vi "S2C_IMAGE_Proc_PassFail.vi"(8 "Error In":errorcluster, 11 "ImagePath":path) -> (0 "Error Out":errorcluster, 3 "Result":string)   [LabVIEW 2015]
panel:
  in  "Submit":bool
  in  "Blemesh":bool
  in  "Chip":bool
  in  "Dent":bool
  in  "Scratch":bool
  out "Image":picture
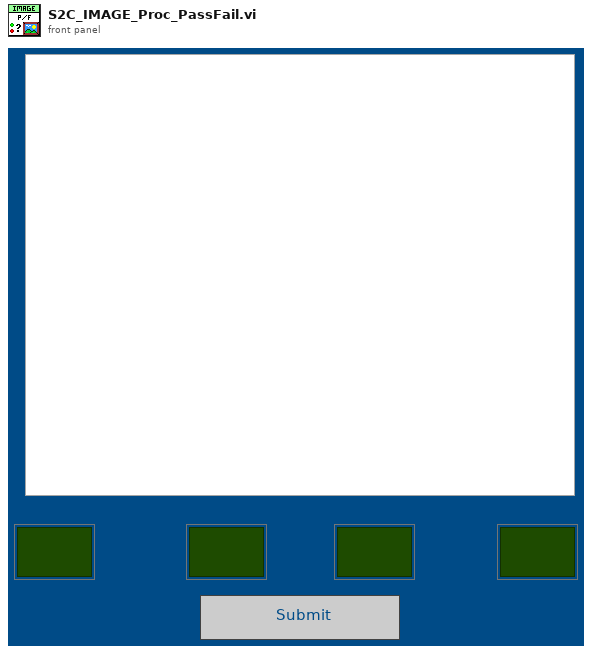
[diagram p1: front panel]
types:
  T1 = cluster{"Left":i16, "Top":i16, "Right":i16, "Bottom":i16}
  T2 = enum32{"Invalid", "Standard", "Closed", "Hidden", "Minimized", "Maximized"}
  T3 = typedef "imagedata.ctl" = cluster{"image type":i32, "image depth":i32, "image":u8[], "mask":u8[], "colors":u32[], "Rectangle":cluster{"left":i16, "top":i16, "right":i16, "bottom":i16}}
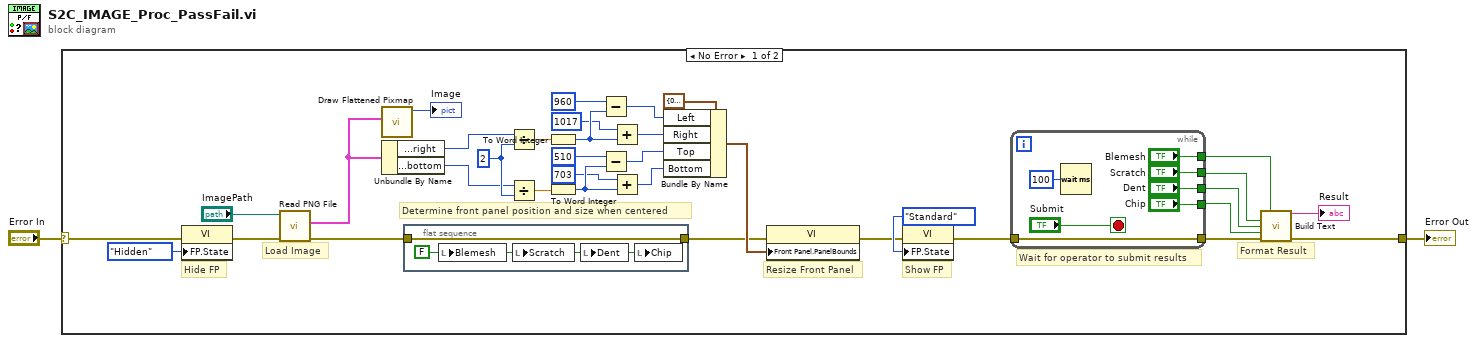
[diagram p0: block diagram]
diagram:
  n1 = case shown="No Error" "Error In" {
    selector: "Error In" -> [w34 w47]
    tunnel: [w26 w47] -> w1
    frame No Error {
      w28 = i16 2 ("y")
      # "Format Result"
      # "Show FP"
      # "Resize Front Panel"
      # "Determine front panel position and size when centered"
      # "Hide FP"
      # "Wait for operator to submit results"
      # "Load Image"
      n2 = property class="VI"(error in=w34, "FP.State"=T2."Hidden" ("Front Panel Window:State")) -> (error out=w32:errorcluster)  [unwired: 1 in, 1 out]
      n3 = call <vilib>:"Read PNG File.vi"("error in (no error)"=w32, "path to PNG file"="ImagePath") -> ("error out"=w4:errorcluster, "image data"=w35:T3)  [unwired: 7 in, 1 out]
      n4 = call <vilib>:"Draw Flattened Pixmap.vi"("image data"=w35) -> ("new picture"=→"Image":picture)  [unwired: 8 in]
      n5 = Unbundle By Name(w35) -> ("Rectangle.right"=w7:i16, "Rectangle.bottom"=w6:i16)
      n6 = flat-sequence {
        tunnel: w4 -> [w39]
        tunnel: [w39] -> w3
        frame #0 {
          w38 = FALSE ("Blemesh")
          n7 = local write "Blemesh"(w38) -> ()
          n8 = local write "Scratch"(w38) -> ()
          n9 = local write "Dent"(w38) -> ()
          n10 = local write "Chip"(w38) -> ()
        }
      }
      n11 = Divide(x=w7, y=w28) -> (x/y=w9:dbl)
      n12 = Divide(x=w6, y=w28) -> (x/y=w8:dbl)
      n13 = To Word Integer(number=w9) -> (16bit integer=w19:i16)
      n14 = To Word Integer(number=w8) -> (16bit integer=w18:i16)
      n15 = Subtract(x=i16 960, y=w19) -> (x-y=w16:i16)
      n16 = Subtract(x=i16 510, y=w18) -> (x-y=w14:i16)
      n17 = Add(x=i16 1017, y=w19) -> (x+y=w15:i16)
      n18 = Add(x=i16 703, y=w18) -> (x+y=w13:i16)
      n19 = Bundle By Name(cluster=T1 {"Left"=0, "Top"=0, "Right"=0, "Bottom"=0} ("Front Panel Window:Panel Bounds"), "Left"=w16, "Right"=w15, "Top"=w14, "Bottom"=w13) -> (w5:T1)
      n20 = property class="VI"(error in=w3, "Front Panel.PanelBounds"=w5) -> (error out=w30:errorcluster)  [unwired: 1 in, 1 out]
      n21 = property class="VI"(error in=w30, "FP.State"=T2."Standard" ("Front Panel Window:State")) -> (error out=w29:errorcluster)  [unwired: 1 in, 1 out]
      n22 = while {
        tunnel: w29 -> [w46]
        tunnel: [w46] -> w27
        tunnel: ["Blemesh"] -> w25
        tunnel: ["Scratch"] -> w24
        tunnel: ["Dent"] -> w23
        tunnel: ["Chip"] -> w22
        stop <- "Submit" stop-if-true
        n23 = Wait (ms)(milliseconds to wait=u32 100) -> ()  [unwired: 1 out]
      }
      n24 = call "Build Text"("Blemish"=w25, "Scratch"=w24, "Dent"=w23, "Chip"=w22, "error in (no error)"=w27) -> ("Result"=→"Result":string, "error out"=w26:errorcluster)  [unwired: 9 in]
    }
    frame Error {
    }
  }
  "Error Out" <- w1
